vi "Root ID.vi"(4 "Resource in":refnum<class "Resource.lvclass">) -> (7 "Root ID":string)   [LabVIEW 2024, in "CTI.lvlib" / "Resource.lvclass"]
uses:
  Resource.lvclass
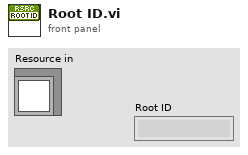
[diagram p1: front panel]
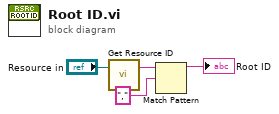
[diagram p0: block diagram]
diagram:
  n1 = call-dynamic "Get Resource ID.vi"("Resource in"="Resource in") -> ("Resource ID"=w3:string)  [unwired: 6 in]
  n2 = Match Pattern(string=w3, regular expression=",") -> (before substring=→"Root ID":string)  [unwired: 1 in, 3 out]
